vi "Byte Buffer.Set Buffer Size.vi"(8 "error in (no error)":errorcluster, 10 "buffer size":u64, 11 "Byte Buffer in":refnum<class "Byte Buffer.lvclass">) -> (0 "error out":errorcluster, 3 "Byte Buffer out":refnum<class "Byte Buffer.lvclass">)   [LabVIEW 2016, in "VeriStand Data.lvlib" / "Byte Buffer.lvclass"]
uses:
  Byte Buffer.lvclass
  Byte Buffer.lvclass/Byte Buffer.ctl
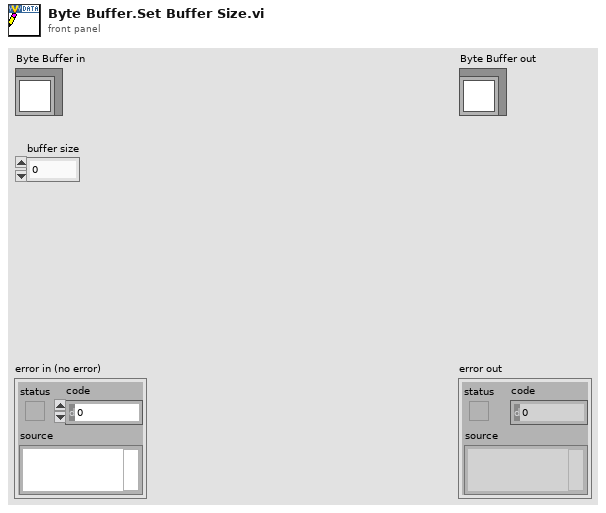
[diagram p1: front panel]
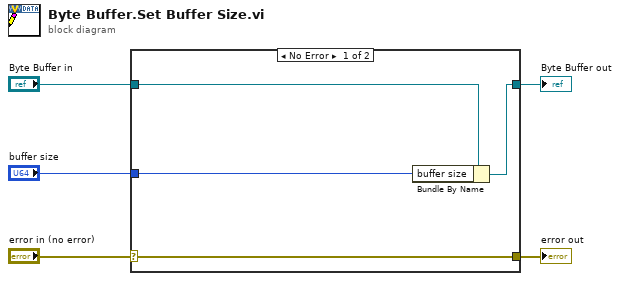
[diagram p0: block diagram]
diagram:
  n1 = case shown="No Error" "error in (no error)" {
    selector: "error in (no error)" -> [w9 w10]
    tunnel: [w9 w10] -> w4
    tunnel: [w7 w11] -> w2
    tunnel: "Byte Buffer in" -> [w8 w11]
    tunnel: "buffer size" -> [w6 _]
    frame No Error {
      n2 = Bundle By Name(cluster=w8, "buffer size"=w6) -> (w7:refnum<class "Byte Buffer.lvclass">)
    }
    frame Error {
    }
  }
  "error out" <- w4
  "Byte Buffer out" <- w2
